vi "Parse_Quotes.vi"(8 "error in (no error)":errorcluster, 11 "JSON String In":string) -> (0 "error out":errorcluster, 1 "Found?":bool, 2 "Examples":string, 3 "JSON String Out":string)   [LabVIEW 2018, in "MerriamWebsterJSON.lvlib"]
uses:
  MerriamWebsterJSON.lvlib
  <vilib>/LVH/i3 JSON/JSON Parsing/Get Array Value at Index Files/Get Array Value at Index - Object.vi
  <vilib>/LVH/i3 JSON/JSON Parsing/Get Object Parameter Files/Get Object Parameter - Object.vi
  <vilib>/LVH/i3 JSON/JSON Parsing/Get Object Parameter Files/Get Object Parameter - String.vi
  <vilib>/LVH/i3 JSON/i3-json.lvlib
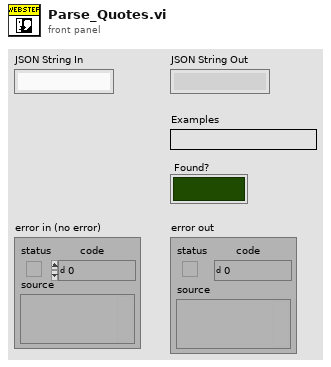
[diagram p1: front panel]
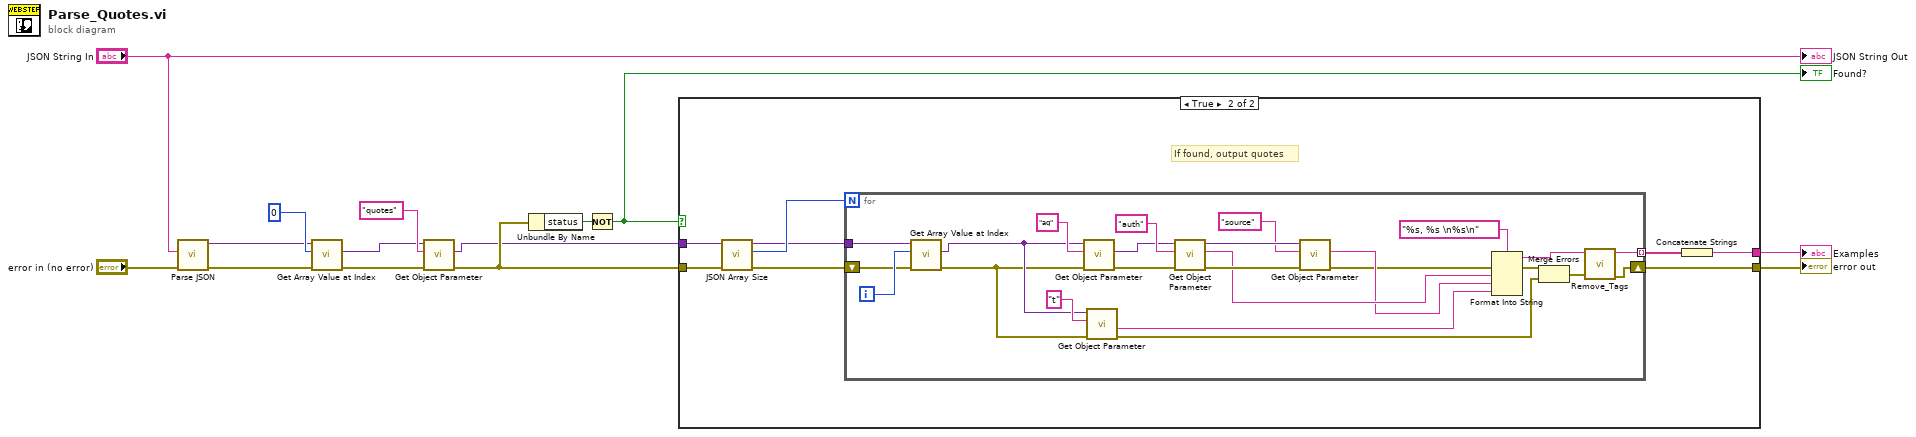
[diagram p0: block diagram]
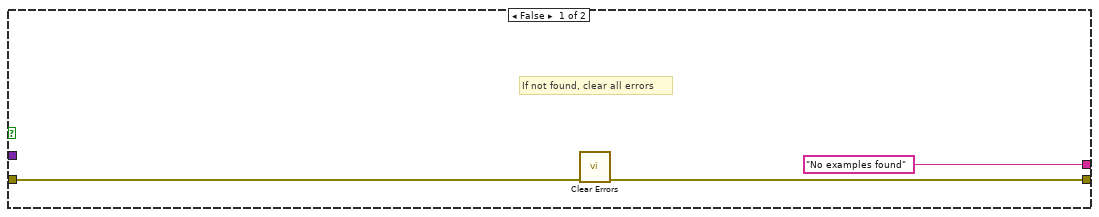
[diagram p2: hidden frame]
diagram:
  n1 = call <vilib>:"Parse JSON.vi"("error in (no error)"="error in (no error)", "JSON String"="JSON String In") -> ("error out"=w13:errorcluster, "JSON Tree"=w11:variant)  [unwired: 6 in, 2 out]
  n2 = call-poly <vilib>:"Get Array Value at Index.vi"("error in (no error)"=w13, "Index"=0, "JSON Tree In (JSON Array)"=w11) -> ("error out"=w10:errorcluster, "JSON Object"=w4:variant)  [unwired: 5 in, 2 out]
  n3 = call-poly <vilib>:"Get Object Parameter.vi"("error in (no error)"=w10, "Parameter Name"="quotes", "JSON Tree In (JSON Object)"=w4) -> ("error out"=w6:errorcluster, "JSON Object"=w5:variant)  [unwired: 5 in, 2 out]
  n4 = Unbundle By Name(w6) -> ("status"=w8:bool)
  n5 = Not(x=w8) -> (.not. x?=w7:bool)
  "Found?" <- w7
  n6 = case shown="True" w7 {
    tunnel: w6 -> [w17 w25]
    tunnel: w5 -> [_ w24]
    tunnel: ["No examples found" ("String Value") w19] -> w3
    tunnel: [w15 w18] -> w2
    frame False {
      # "If not found, clear all errors"
      n7 = call <vilib>:"Clear Errors.vi"("error in (no error)"=w17) -> ("error out"=w15:errorcluster)  [unwired: 5 in, 1 out]
    }
    frame True {
      # "If found, output quotes"
      n8 = call <vilib>:"JSON Array Size.vi"("error in (no error)"=w25, "JSON Tree In (JSON Array)"=w24) -> ("error out"=w21:errorcluster, "Array Size"=w23:i32, "JSON Tree Passthrough (JSON Array)"=w22:variant)  [unwired: 7 in]
      n9 = for {
        N: w23 -> [_]
        tunnel: w22 -> [w39]
        tunnel: [w31] -> w20 mode=indexing
        shift-right: [w26] -> w18
        shift-left: w21 -> [w38]
        i -> [w41]
        n10 = call-poly <vilib>:"Get Array Value at Index.vi"("error in (no error)"=w38, "Index"=w41, "JSON Tree In (JSON Array)"=w39) -> ("error out"=w37:errorcluster, "JSON Object"=w40:variant)  [unwired: 5 in, 2 out]
        n11 = call-poly <vilib>:"Get Object Parameter.vi"("error in (no error)"=w37, "Parameter Name"="aq", "JSON Tree In (JSON Object)"=w40) -> ("error out"=w43:errorcluster, "JSON Object"=w44:variant)  [unwired: 5 in, 2 out]
        n12 = call-poly <vilib>:"Get Object Parameter.vi"("error in (no error)"=w37, "Parameter Name"="t", "JSON Tree In (JSON Object)"=w40) -> ("error out"=w28:errorcluster, "String Value"=w33:string)  [unwired: 5 in, 2 out]
        n13 = call-poly <vilib>:"Get Object Parameter.vi"("error in (no error)"=w43, "Parameter Name"="auth", "JSON Tree In (JSON Object)"=w44) -> ("error out"=w46:errorcluster, "String Value"=w35:string, "JSON Tree Out Passthrough"=w48:variant)  [unwired: 5 in, 1 out]
        n14 = call-poly <vilib>:"Get Object Parameter.vi"("error in (no error)"=w46, "Parameter Name"="source", "JSON Tree In (JSON Object)"=w48) -> ("error out"=w30:errorcluster, "String Value"=w34:string)  [unwired: 5 in, 2 out]
        n15 = Format Into String(format string="%s, %s \n%s\n", error in=w30, w35, w34, w33) -> (resulting string=w32:string, error out=w29:errorcluster)  [unwired: 1 in]
        n16 = Merge Errors(w29, w28) -> (w27:errorcluster)
        n17 = call "Remove_Tags.vi"("error in (no error)"=w27, "Input String"=w32) -> ("error out"=w26:errorcluster, "Output String"=w31:string)  [unwired: 8 in]
      }
      n18 = Concatenate Strings(w20) -> (w19:string)
    }
  }
  "error out" <- w2
  "Examples" <- w3
  "JSON String Out" <- "JSON String In"
